vi "Comm Disconnect.vi"(8 "error in (no error)":errorcluster, 11 "niDTS Comm Telnet in":refnum<class "niDTS Comm Telnet.lvclass">) -> (0 "error out":errorcluster, 3 "niDTS Comm Telnet out":refnum<class "niDTS Comm Telnet.lvclass">)   [LabVIEW 2015, in "niDTS CommLib.lvlib" / "niDTS Comm Telnet.lvclass"]
uses:
  niDTS Comm Telnet.lvclass
  Utility/telnet/NI_InternetTK_Core_VIs.lvlib
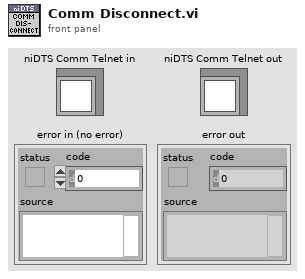
[diagram p1: front panel]
types:
  T1 = typedef "Telnet Session.ctl" = refnum<k1>
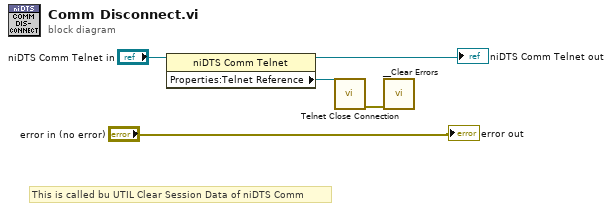
[diagram p0: block diagram]
diagram:
  # "This is called bu UTIL Clear Session Data of niDTS Comm"
  n1 = property class="niDTS Comm Telnet"(reference="niDTS Comm Telnet in") -> (reference out=→"niDTS Comm Telnet out":refnum<class "niDTS Comm Telnet.lvclass">, "Properties:Telnet Reference"=w3:T1)  [unwired: 1 in, 1 out]
  n2 = call "Telnet Close Connection.vi"("telnet connection"=w3) -> ("error out"=w4:errorcluster)  [unwired: 9 in, 1 out]
  n3 = call "__Clear Errors.vi"("error in (no error)"=w4) -> ()  [unwired: 5 in, 2 out]
  "error out" <- "error in (no error)"
